vi "Do.vi"(8 "error in (no error)":cluster{"状态":bool, "代码":i32, "源":string} caption="错误输入（无错误）", 10 "操作者输入":refnum<class "Actor.lvclass">, 11 "?":refnum<class "Swap Controllers Msg.lvclass">) -> (0 "error out":cluster{"状态":bool, "代码":i32, "源":string} caption="错误输出", 2 "操作者输出":refnum<class "Actor.lvclass">)   [LabVIEW 2015, in "Air Cooler Application.lvlib" / "Swap Controllers Msg.lvclass"]
uses:
  Swap Controllers Msg.lvclass
  <vilib>/ActorFramework/Actor/Actor.lvclass
  Air Cooler Application/Air Cooler Application.lvclass
  Swap Controllers Msg.lvclass/Swap Controllers Msg.ctl
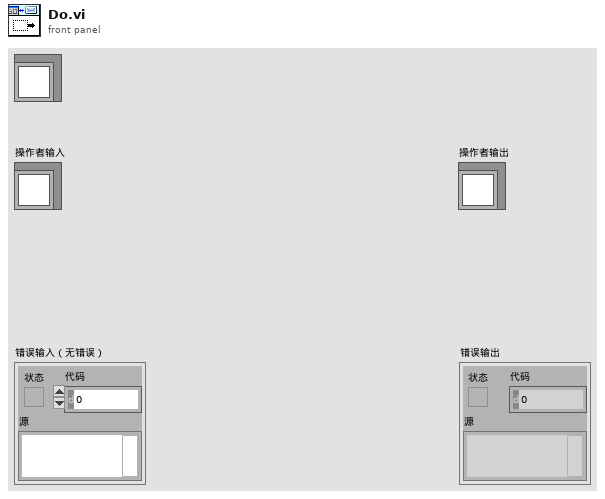
[diagram p1: front panel]
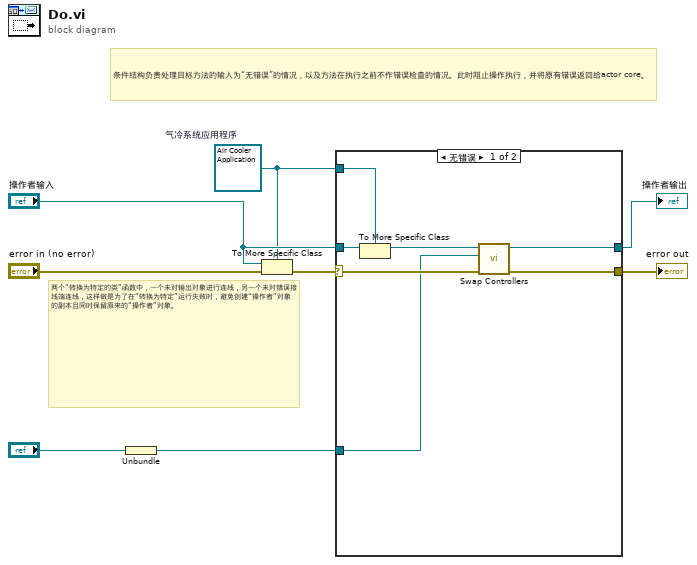
[diagram p0: block diagram]
diagram:
  w2 = refnum<class "Air Cooler Application.lvclass"> refnum  # 气冷系统应用程序
  # "两个“转换为特定的类”函数中，一个未对输出对象进行连线，另一个未对错误接线端连线，这样做是为了在“转换为特定”运行失败时，避免创建“操作者”对象的副本且同时保留原来的“操作者”对象。"
  # "条件结构负责处理目标方法的输入为“无错误”的情况，以及方法在执行之前不作错误检查的情况。此时阻止操作执行，并将原有错误返回给actor core。"
  n1 = Unbundle("?") -> (w1:refnum<class "Cooler Controller.lvclass">)
  n2 = To More Specific Class(target class=w2, reference="操作者输入", error in="error in (no error)") -> (error out=w6:errorcluster)  [unwired: 1 out]
  n3 = case shown="无错误" w6 {
    selector: w6 -> [w13 w17]
    tunnel: [w15 w17] -> w5
    tunnel: [w14 w16] -> w4
    tunnel: "操作者输入" -> [w12 w16]
    tunnel: w2 -> [w11 _]
    tunnel: w1 -> [w9 _]
    frame No Error {
      n4 = To More Specific Class(target class=w11, reference=w12) -> (specific class reference=w10:refnum<class "Air Cooler Application.lvclass">)  [unwired: 1 in, 1 out]
      n5 = call "Swap Controllers.vi"("error in (no error)"=w13, "冷却器控制器"=w9, "气冷系统应用程序输入"=w10) -> ("error out"=w15:cluster{"状态":bool, "代码":i32, "源":string}, "气冷系统应用程序输出"=w14:refnum<class "Air Cooler Application.lvclass">)  [unwired: 7 in]
    }
    frame Error {
      # "如类型检查失败，则再次将原对象传出。"
    }
  }
  "error out" <- w5
  "操作者输出" <- w4
